vi "FPGA_Y value calulate.vi"(9 "上限":i16, 10 "Y Offset":i16, 11 "Y Amplitude":fxp<+,16,0> format="%.16g") -> (3 "数值输入控件":i16)   [LabVIEW 2015]
uses:
  <vilib>/rvi/FXPMathLib/FxpMul/XNode/nifxpmath_Multiplier.xnode
  <vilib>/rvi/FXPMathLib/sim/FxpSim.dll
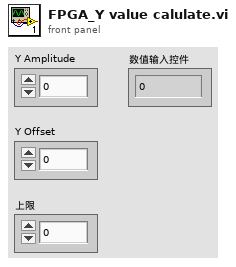
[diagram p1: front panel]
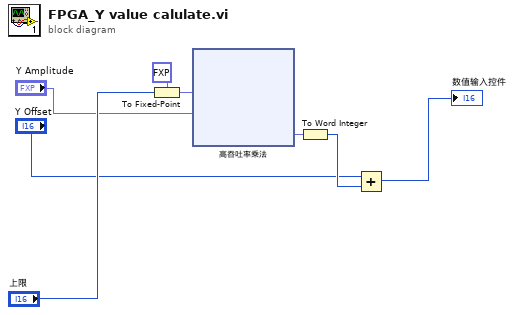
[diagram p0: block diagram]
diagram:
  n1 = To Fixed-Point(fixed-point type=fxp<+/-,17,17> 0.0 ("定点"), number="上限") -> (fixed-point=w4:fxp<+/-,17,17>)
  n2 = xnode ("高吞吐率乘法")("x"=w4, "y"="Y Amplitude") -> ("x*y"=w3:fxp<+/-,16,16>)
  n3 = To Word Integer(number=w3) -> (16bit integer=w6:i16)
  n4 = Add(x="Y Offset", y=w6) -> (x+y=→"数值输入控件":i16)
